vi "TreeNode Get Segment Limits.vi"(8 "error in (no error)":errorcluster, 10 "segmentIdxIn":i32, 11 "TreeNode DVR in":refnum<data-value>) -> (0 "error out":errorcluster, 1 "End Segment":i64, 2 "Start Segment":i64 format="%.4f", 3 "TreeNode DVR out":refnum<data-value>)   [LabVIEW 2015, in "MDSplus.lvlib"]
uses:
  <vilib>/MDSplus/Library/MDSplus.lvlib
  <vilib>/MDSplus/Classes/Data_Class/TreeNode_Class/TreeNode.lvclass
  <vilib>/MDSplus/Classes/Data_Class/Data.lvclass
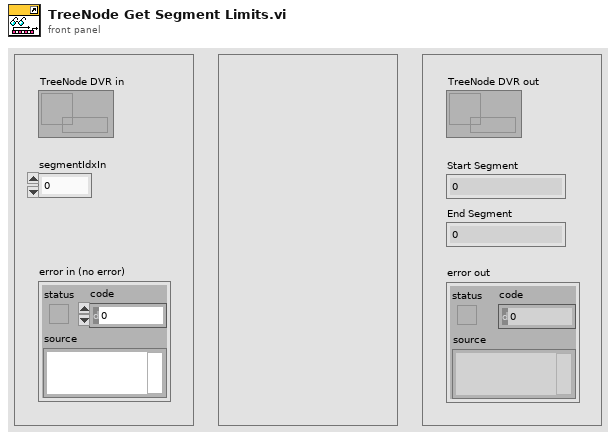
[diagram p1: front panel]
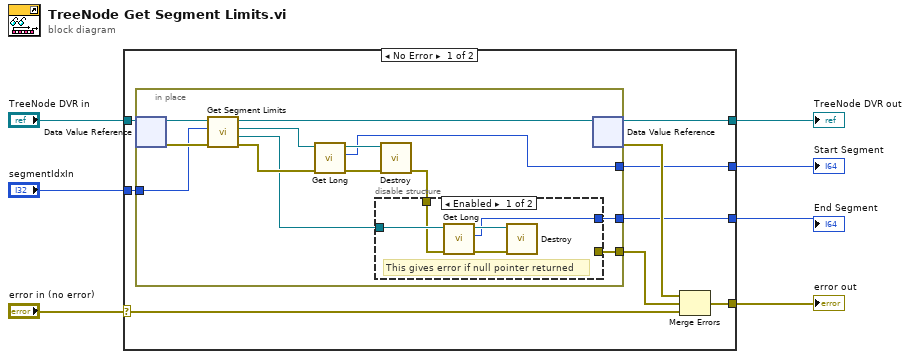
[diagram p0: block diagram]
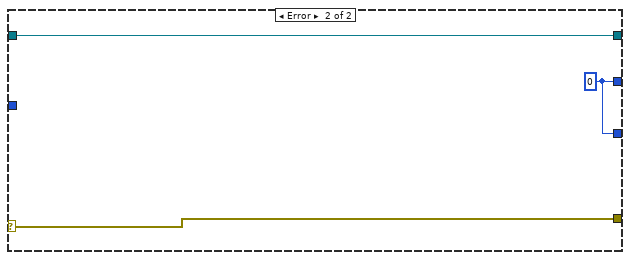
[diagram p3: hidden frame]
diagram:
  n1 = case shown="No Error" "error in (no error)" {
    selector: "error in (no error)" -> [w15 w38]
    tunnel: "TreeNode DVR in" -> [w16 w37]
    tunnel: [w12 w38] -> w7
    tunnel: [w13 w37] -> w4
    tunnel: [w10 w36] -> w3
    tunnel: [w9 w36] -> w2
    tunnel: "segmentIdxIn" -> [w8 _]
    frame No Error {
      n2 = in-place {
        in-place-border: [w17] -> w11
        in-place-border: [w21] -> w10
        in-place-border: [w19] -> w9
        in-place-border: w8 -> [w18]
        n3 = in-place-dvr #1(w16) -> (w29:refnum<class "TreeNode.lvclass">, w28:errorcluster)
        n4 = call-dynamic "Get Segment Limits.vi"("error in (no error)"=w28, "segmentIdxIn"=w18, "TreeNode in"=w29) -> ("error out"=w25:errorcluster, "End Data out"=w24:refnum<class "Data.lvclass">, "Start Data out"=w26:refnum<class "Data.lvclass">, "TreeNode out"=w27:refnum<class "TreeNode.lvclass">)  [unwired: 5 in]
        n5 = call-dynamic "Get Long.vi"("error in (no error)"=w25, "Data in"=w26) -> ("error out"=w22:errorcluster, "I64 out"=w21:i64, "Data out"=w23:refnum<class "Data.lvclass">)  [unwired: 7 in]
        n6 = call-dynamic "Destroy.vi"("error in (no error)"=w22, "Data in"=w23) -> ("error out"=w20:errorcluster)  [unwired: 9 in]
        n7 = disable-structure shown="Enabled" {
          disable-tunnel: w24 -> [w34 _]
          disable-tunnel: w20 -> [w33 w35]
          disable-tunnel: [w30 _] -> w19
          disable-tunnel: [_ w35] -> w17
          frame Enabled {
            # "This gives error if null pointer returned"
            n8 = call-dynamic "Get Long.vi"("error in (no error)"=w33, "Data in"=w34) -> ("error out"=w32:errorcluster, "I64 out"=w30:i64, "Data out"=w31:refnum<class "Data.lvclass">)  [unwired: 7 in]
            n9 = call-dynamic "Destroy.vi"("error in (no error)"=w32, "Data in"=w31) -> ()  [unwired: 9 in, 1 out]
          }
          frame Disabled {
          }
        }
        n10 = in-place-dvr #1(w27) -> (w13:refnum<data-value>, w14:errorcluster)
      }
      n11 = Merge Errors(w14, w11, w15) -> (w12:errorcluster)
    }
    frame Error {
      w36 = i64 0 ("I64 out")
    }
  }
  "error out" <- w7
  "TreeNode DVR out" <- w4
  "Start Segment" <- w3
  "End Segment" <- w2
